vi "MiPS_read.vi"(6 "ISOBUS address":T4, 8 "error in":errorcluster, 11 "ref_in":T1) -> (0 "error out":errorcluster, 1 "Voltage":dbl, 2 "Current":dbl, 3 "ref_out":T1, 4 "heater_status":bool, 5 "Persistant Current":dbl, 7 "current_in_range":bool)   [LabVIEW 2019]
uses:
  Mercury iXX Modules/Public/Controls/ISOBus Address.ctl
  Mercury iXX Modules/Public/Controls/Mercury Reference.ctl
  Mercury iXX Modules/Public/Controls/Comms Transport Layer.ctl
  Mercury iXX Modules/Private/Controls/Query Dynamic Reference.ctl
  Mercury iXX Modules/Public/Libraries/Magnet/Signals/Read/Persistant Current (Read).vi
  Mercury iXX Modules/Public/Libraries/Magnet/Signals/Read/Current (Read).vi
  Mercury iXX Modules/Public/Libraries/Magnet/Signals/Read/Voltage (Read).vi
  Mercury iXX Modules/Public/Libraries/Magnet/Signals/Read/Switch Heater Status (Read).vi
  Mercury iXX Modules/Mercury iXX.lvlib
  Mercury iXX Modules/Public/Libraries/Magnet.lvlib
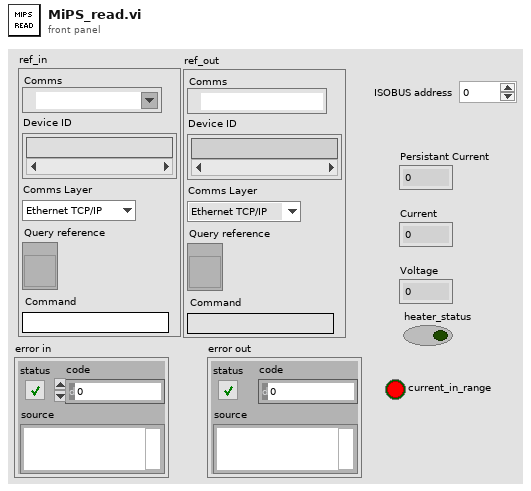
[diagram p1: front panel]
types:
  T1 = typedef "Mercury iXX.lvlib/Mercury Reference.ctl" = cluster{"Comms":refnum<visa-resource-name>, "Device ID":string[], "Comms Layer":T2, "Command":string, "Query reference":T3}
  T2 = typedef "Mercury iXX.lvlib/Comms Transport Layer.ctl" = enum16{"Ethernet TCP/IP", "USB", "ISOBus - RS-232", "GPIB"}
  T3 = typedef "Mercury iXX.lvlib/Query Dynamic Reference.ctl" = refnum<vi>
  T4 = typedef "Mercury iXX.lvlib/ISOBus Address.ctl" = i32
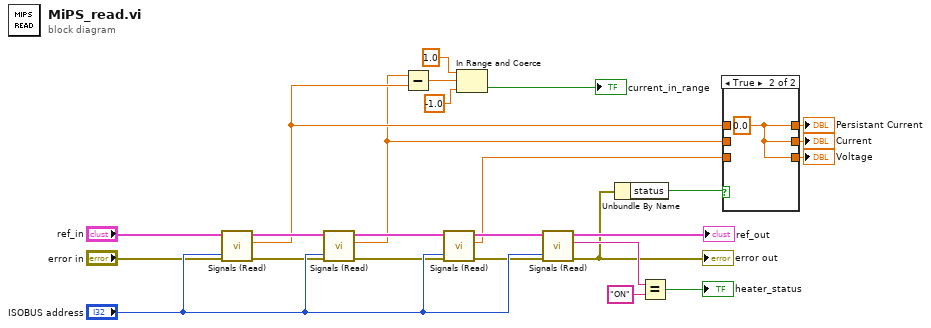
[diagram p0: block diagram]
diagram:
  n1 = call-poly "Signals (Read).vi"("ISOBUS address"="ISOBUS address", "error in"="error in", "Mercury Reference In"="ref_in") -> ("error out"=w20:errorcluster, "Persistant Current"=w5:dbl, "Mercury Reference Out"=w22:T1)  [unwired: 4 in, 2 out]
  n2 = call-poly "Signals (Read).vi"("ISOBUS address"="ISOBUS address", "error in"=w20, "Mercury Reference In"=w22) -> ("error out"=w17:errorcluster, "Current"=w3:dbl, "Mercury Reference Out"=w13:T1)  [unwired: 4 in, 2 out]
  n3 = Subtract(x=w3, y=w5) -> (x-y=w12:dbl)
  n4 = call-poly "Signals (Read).vi"("ISOBUS address"="ISOBUS address", "error in"=w17, "Mercury Reference In"=w13) -> ("error out"=w18:errorcluster, "Voltage"=w1:dbl, "Mercury Reference Out"=w14:T1)  [unwired: 4 in, 2 out]
  n5 = In Range and Coerce(upper limit=1.0, x=w12, lower limit=-1.0) -> (In Range?=→"current_in_range":bool)  [unwired: 1 out]
  n6 = call-poly "Signals (Read).vi"("ISOBUS address"="ISOBUS address", "error in"=w18, "Mercury Reference In"=w14) -> ("error out"=w8:errorcluster, "Switch Heater Status"=w24:string, "Mercury Reference Out"=→"ref_out":T1)  [unwired: 5 in, 1 out]
  "error out" <- w8
  n7 = Unbundle By Name(w8) -> ("status"=w7:bool)
  n8 = Equal?(x=w24, y="ON") -> (x = y?=→"heater_status":bool)
  n9 = case shown="True" w7 {
    tunnel: [w28 w29] -> w6
    tunnel: w5 -> [w28 _]
    tunnel: [w27 w29] -> w4
    tunnel: w3 -> [w27 _]
    tunnel: [w26 w29] -> w2
    tunnel: w1 -> [w26 _]
    frame False {
    }
    frame True {
      w29 = 0.0 ("Persistant Current")
    }
  }
  "Persistant Current" <- w6
  "Current" <- w4
  "Voltage" <- w2
